vi "SinglePatternMatch (SubVI).vi"(6 "Color":u32(colorbox)=16711680, 7 "Group":string, 8 "error in (no error)":errorcluster, 9 "Bounding Box":cluster{"x":sgl, "y":sgl}[](array[cluster]), 10 "Position":cluster{"x":sgl, "y":sgl}, 11 "Refnum in":T1) -> (0 "error out":errorcluster, 3 "Refnum out":T1)   [LabVIEW 2011]
uses:
  <vilib>/vision/Image Controls.llb/IMAQ Image.ctl
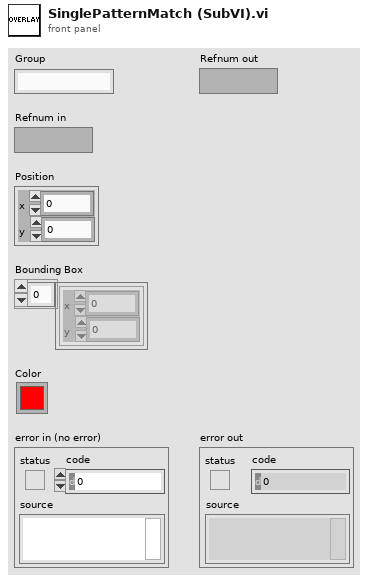
[diagram p1: front panel]
types:
  T1 = typedef "IMAQ Image.ctl" = refnum<image>
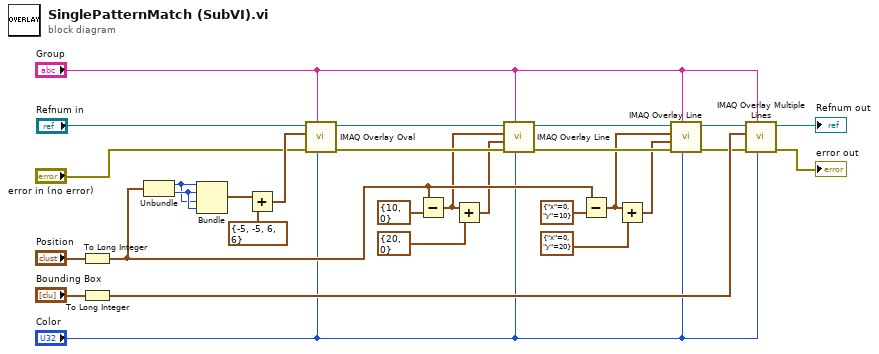
[diagram p0: block diagram]
diagram:
  n1 = To Long Integer(number="Position") -> (32bit integer=w28:cluster{"x":i32, "y":i32})
  n2 = To Long Integer(number="Bounding Box") -> (32bit integer=w29:cluster{"x":i32, "y":i32}[])
  n3 = Unbundle(w28) -> ("x"=w9:i32, "y"=w10:i32)
  n4 = Bundle("x"=w9, "y"=w10, "x"=w9, "y"=w10) -> (w11:cluster{"x":i32, "y":i32, "x":i32, "y":i32})  [unwired: 1 out]
  n5 = Add(x=w11, y=cluster{"y":i32, "x":i32, "y":i32, "x":i32} {"y"=-5, "x"=-5, "y"=6, "x"=6}) -> (x+y=w13:cluster{i32, i32, i32, i32})
  n6 = call "IMAQ Overlay Oval"("Color"="Color", "Group"="Group", "error in (no error)"="error in (no error)", "Bounding Rectangle"=w13, "Image"="Refnum in") -> ("error out"=w23:errorcluster, "Image Out"=w7:T1)  [unwired: 1 in, 4 out]
  n7 = Subtract(x=w28, y=cluster{"x":i32, "y":i32} {"x"=10, "y"=0}) -> (x-y=w15:cluster{"x":i32, "y":i32})
  n8 = Add(x=w15, y=cluster{"x":i32, "y":i32} {"x"=20, "y"=0}) -> (x+y=w17:cluster{"x":i32, "y":i32})
  n9 = call "IMAQ Overlay Line"("Color"="Color", "Group"="Group", "error in (no error)"=w23, "End Point"=w17, "Start Point"=w15, "Image"=w7) -> ("error out"=w24:errorcluster, "Image Out"=w22:T1)  [unwired: 4 out]
  n10 = Subtract(x=w28, y=cluster{"x":i32, "y":i32} {"x"=0, "y"=10}) -> (x-y=w19:cluster{"x":i32, "y":i32})
  n11 = Add(x=w19, y=cluster{"x":i32, "y":i32} {"x"=0, "y"=20}) -> (x+y=w18:cluster{"x":i32, "y":i32})
  n12 = call "IMAQ Overlay Line"("Color"="Color", "Group"="Group", "error in (no error)"=w24, "End Point"=w18, "Start Point"=w19, "Image"=w22) -> ("error out"=w25:errorcluster, "Image Out"=w8:T1)  [unwired: 4 out]
  n13 = call "IMAQ Overlay Multiple Lines"("Color"="Color", "Group"="Group", "error in (no error)"=w25, "Line End Points"=w29, "Image"=w8) -> ("error out"=→"error out":errorcluster, "Image Out"=→"Refnum out":T1)  [unwired: 1 in, 4 out]
